vi "4Pi Obj Lock - 2 Values Organize Plot Data.vi"(0 "Target 01":dbl, 2 "Value Limit":dbl, 5 "Target 02":dbl, 9 "Current 01":dbl, 11 "Current 02":dbl) -> (8 "Plot Data":T1)   [LabVIEW 2016]
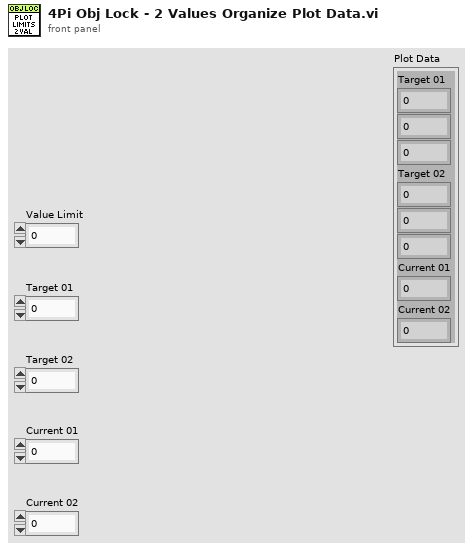
[diagram p1: front panel]
types:
  T1 = cluster{"Target 01":dbl, dbl, dbl, "Target 02":dbl, dbl, dbl, "Current 01":dbl, "Current 02":dbl}
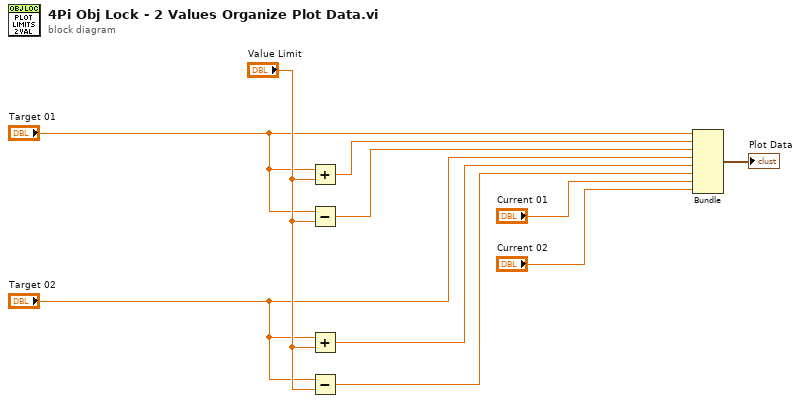
[diagram p0: block diagram]
diagram:
  n1 = Add(x="Target 01", y="Value Limit") -> (x+y=w8:dbl)
  n2 = Subtract(x="Target 01", y="Value Limit") -> (x-y=w7:dbl)
  n3 = Add(x="Target 02", y="Value Limit") -> (x+y=w5:dbl)
  n4 = Subtract(x="Target 02", y="Value Limit") -> (x-y=w4:dbl)
  n5 = Bundle("Target 01"="Target 01", w8, w7, "Target 02"="Target 02", w5, w4, "Current 01"="Current 01", "Current 02"="Current 02") -> (→"Plot Data":T1)  [unwired: 1 in]
